vi "VALVE_wait_for_task_START.vi"(1 "error in":errorcluster) -> (0 "error out":errorcluster)   [LabVIEW 2015]
uses:
  GLOBAL/Global_VALVE.vi
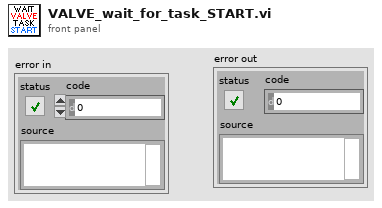
[diagram p1: front panel]
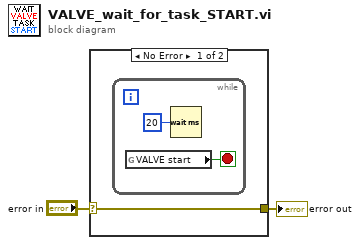
[diagram p0: block diagram]
diagram:
  n1 = case shown="No Error" "error in" {
    selector: "error in" -> [w3 w6]
    tunnel: [w3 w6] -> w1
    frame No Error {
      n2 = while {
        stop <- w5 stop-if-true
        n3 = global read "Global_VALVE.vi" "VALVE start"() -> (w5:bool)
        n4 = Wait (ms)(milliseconds to wait=u32 20) -> ()  [unwired: 1 out]
      }
    }
    frame Error {
    }
  }
  "error out" <- w1
